vi "2D_density_plot_test.vi"() -> ()   [LabVIEW 2018]
uses:
  <vilib>/Heliosphere Research LLC/Advanced Plotting Toolkit/api_plotting/ContourFilledProperties.ctl
  <vilib>/Heliosphere Research LLC/Advanced Plotting Toolkit/properties/Colormap.ctl
  <vilib>/Heliosphere Research LLC/Advanced Plotting Toolkit/properties/Colormap_Map.ctl
  <vilib>/Heliosphere Research LLC/Advanced Plotting Toolkit/properties/Colormap_Scaling.ctl
  <vilib>/Heliosphere Research LLC/Advanced Plotting Toolkit/properties/Display.ctl
  <vilib>/Heliosphere Research LLC/Advanced Plotting Toolkit/api_plotting/ContourRange.ctl
  <vilib>/Heliosphere Research LLC/Advanced Plotting Toolkit/api_core/NewPlotType.ctl
  <vilib>/Heliosphere Research LLC/Advanced Plotting Toolkit/api_core/NewPlotScales.ctl
  <vilib>/Heliosphere Research LLC/Advanced Plotting Toolkit/api_plotting/ContourFilled_Automatic.vi
  <vilib>/Heliosphere Research LLC/Advanced Plotting Toolkit/Advanced Plotting Toolkit.lvlib
panel:
  in  "Contour Range":T1={"Min Level"=nan, "Max Level"=nan}
  in  "Log-transform?":bool=TRUE
  in  "Properties":T2={"Colormap"={"Map"=enum."Automatic", "Value Min"=nan, "Value Max"=nan, "Scaling"=enum."Default", "Reverse"=FALSE}, "Display"={"Alpha"=nan, "Z Order"=nan}}
  out "Picture":picture
  out "Image Display":T7(plugin-control)
  in  "Python file path":path
  out "alpha":dbl[](array[numeric])
  out "Y coord":dbl[](array[numeric])
  out "X coord":dbl[](array[numeric])
  out "error out":errorcluster
  in  "create index file? (T)":bool
  in  "File path":path
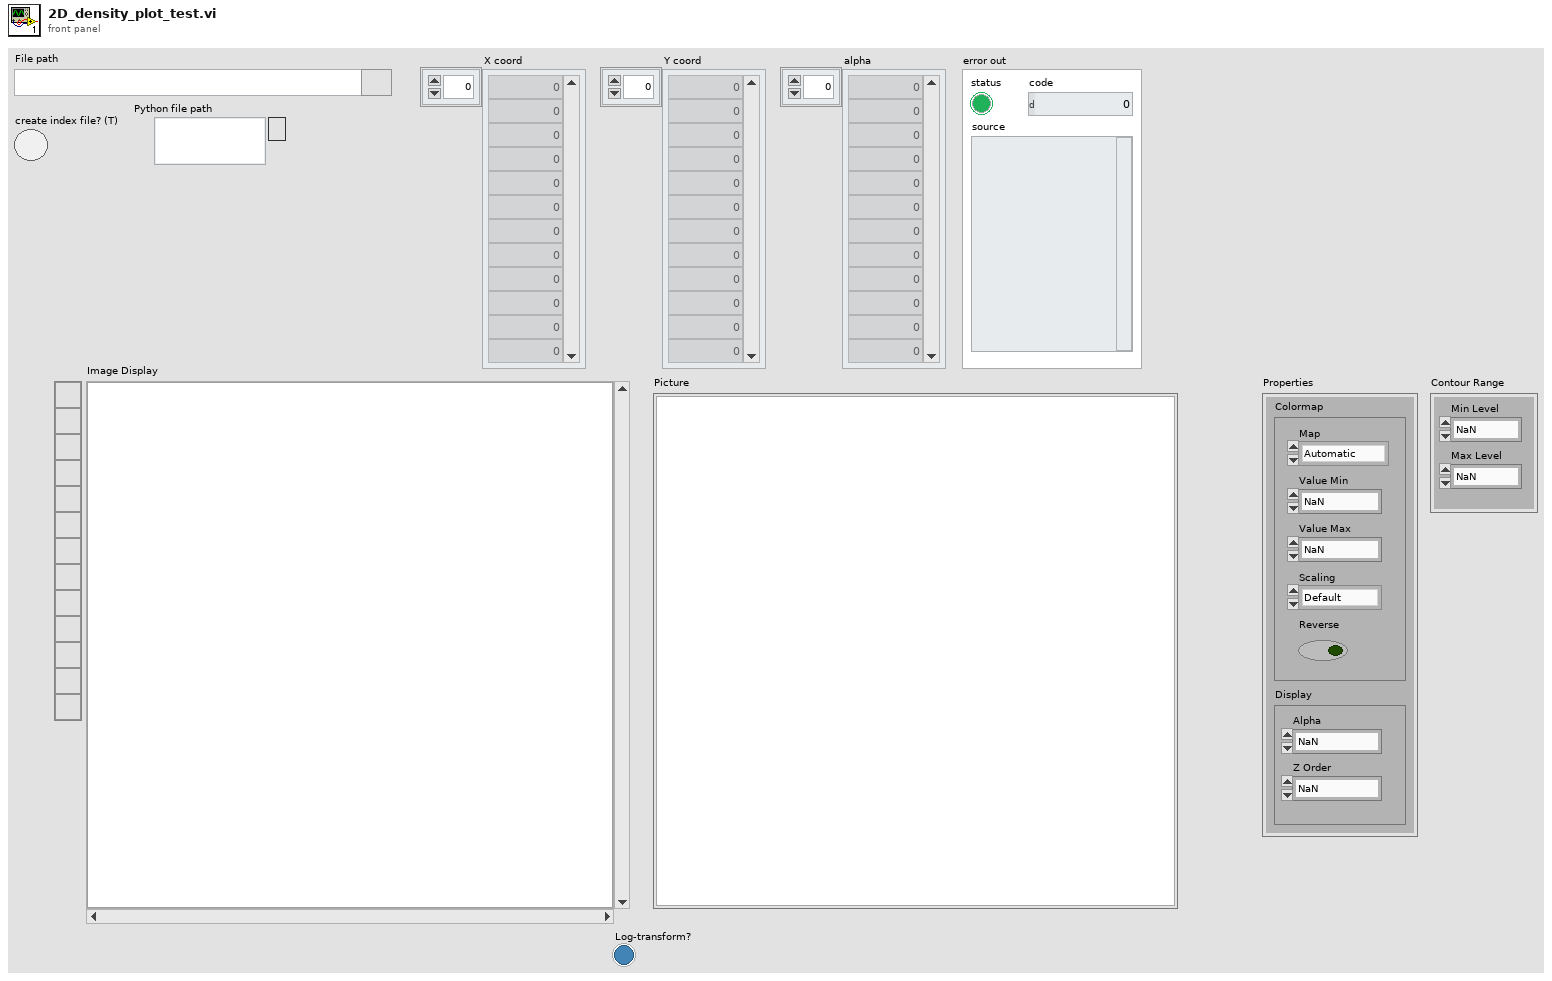
[diagram p1: front panel]
types:
  T1 = typedef "Advanced Plotting Toolkit.lvlib/ContourRange.ctl" = cluster{"Min Level":dbl, "Max Level":dbl}
  T2 = typedef "Advanced Plotting Toolkit.lvlib/ContourFilledProperties.ctl" = cluster{"Colormap":T3, "Display":T6}
  T3 = typedef "Advanced Plotting Toolkit.lvlib/Colormap.ctl" = cluster{"Map":T4, "Value Min":dbl, "Value Max":dbl, "Scaling":T5, "Reverse":bool}
  T4 = typedef "Advanced Plotting Toolkit.lvlib/Colormap_Map.ctl" = enum16{"Automatic", "Rainbow", "Hot and Cold", "White-Black", "White-Blue", "White-Green", "White-Red", "Fire", "Water", "Earth", "Air", "Pastel", "Banded", "Stepped"}
  T5 = typedef "Advanced Plotting Toolkit.lvlib/Colormap_Scaling.ctl" = enum16{"Default"}
  T6 = typedef "Advanced Plotting Toolkit.lvlib/Display.ctl" = cluster{"Alpha":dbl, "Z Order":dbl}
  T7 = typedef "IMAQ Image.ctl" = refnum<image>
  T8 = typedef "Advanced Plotting Toolkit.lvlib/NewPlotScales.ctl" = enum16{"Default", "Linear", "Log", "Symlog"}
  T9 = typedef "Advanced Plotting Toolkit.lvlib/NewPlotType.ctl" = enum16{"Rectangular Axes", "Polar Axes"}
  T10 = typedef "Image Type" = u32
  T11 = enum16{"big-endian, network order", "native, host order", "little-endian"}
  T12 = enum16{"open", "open or create", "create or replace", "create", "open (read-only)"}
  T13 = typedef "Advanced Plotting Toolkit.lvlib/PlotID.ctl" = i32
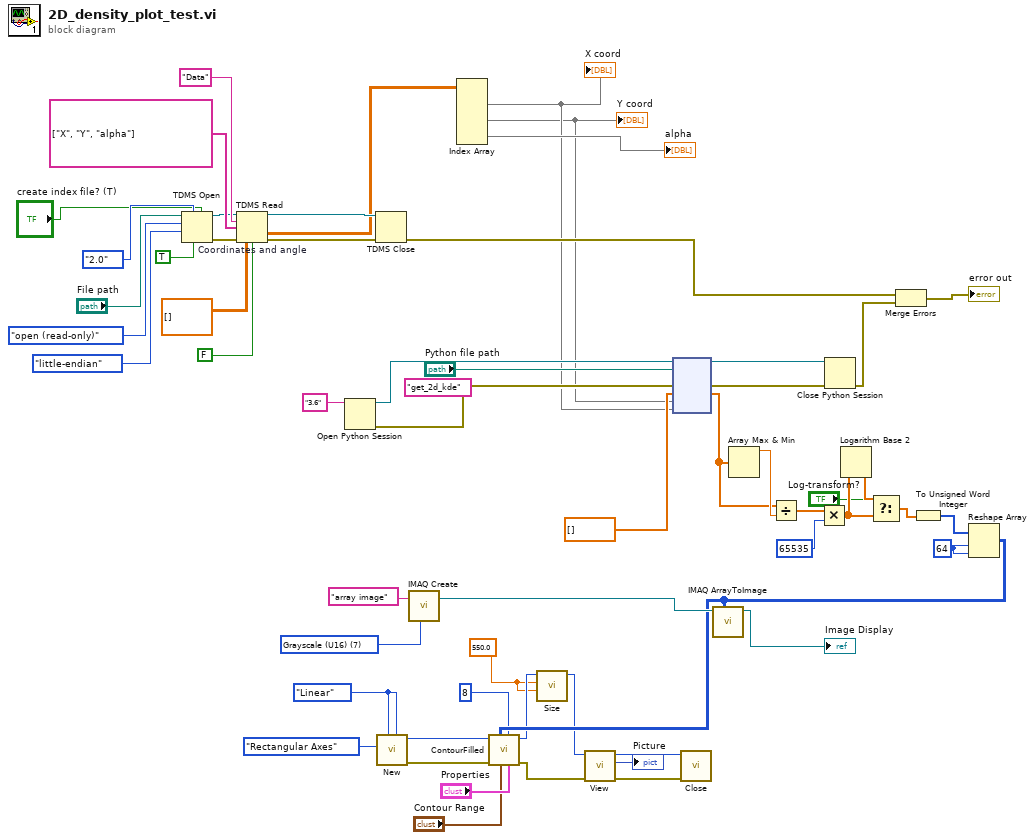
[diagram p0: block diagram]
diagram:
  w6 = 550.0 ("Width (pixels)")
  w18 = NewPlotScales."Linear" ("X Axis Scale")
  w29 = T10 7 items=["Grayscale (U8)", "Grayscale (I16)", "Grayscale (SGL)", "Complex (CSG)", "RGB (U32)", "HSL (U32)", "RGB (U64)", "Grayscale (U16)"] ("Image Type")
  w31 = 64 ("dimension size")
  n1 = TDMS Open(5:"create index file? (T)", 6:TRUE ("disable buffering? (T)"), 7:enum16{"1.0", "2.0"}."2.0" ("file format version (2.0)"), 9:T11."little-endian" ("byte order (2:little-endian)"), 10:T12."open (read-only)" ("operation (0:open)"), 11:"File path") -> (0:w47:errorcluster, 3:w48:refnum<k34>)  [unwired: 1 in]
  n2 = TDMS Read "Coordinates and angle"(0:w48, 5:"Data" ("group name in"), 7:string[] ["X", "Y", "alpha"] ("Columns Names"), 11:w47, 12:dbl[][] [], 13:FALSE ("return channels in file order? (F)")) -> (4:w46:refnum<k34>, 10:w43:dbl[][], 15:w45:errorcluster)  [unwired: 2 in, 3 out]
  n3 = Open Python Session(python version="3.6" ("Python version")) -> (session out=w42:refnum<k35>, error out=w40:errorcluster)  [unwired: 2 in]
  n4 = TDMS Close(8:w45, 11:w46) -> (0:w44:errorcluster)  [unwired: 1 out]
  n5 = call <vilib>:"New.vi"("Y Axis Scale"=w18, "X Axis Scale"=w18, "Plot Type"=NewPlotType."Rectangular Axes") -> ("error out"=w16:errorcluster, "Plot ID"=w17:T13)  [unwired: 7 in]
  n6 = call "IMAQ Create"("Image Name"="array image", "Image Type"=w29) -> ("New Image"=w26:T7)  [unwired: 3 in, 1 out]
  n7 = Index Array(array=w43) -> (element #1=w21:dbl[], element #2=w20:dbl[], element #3=→"alpha":dbl[])  [unwired: 6 in]
  "X coord" <- w21
  "Y coord" <- w20
  n8 = node(w42, "Python file path", "get_2d_kde" ("function name"), w40, dbl[] [], w20, w21) -> (w38:refnum<k35>, w37:errorcluster, w23:dbl[])  [unwired: 2 in, 2 out]
  n9 = Array Max & Min(array=w23) -> (max value=w28:dbl)  [unwired: 3 out]
  n10 = Divide(x=w23, y=w28) -> (x/y=w22:dbl[])
  n11 = Multiply(x=w22, y=65535 ("dimension size")) -> (x*y=w4:dbl[])
  n12 = Close Python Session(session in=w38, error in=w37) -> (11:w35:errorcluster)
  n13 = Logarithm Base 2(1:w4) -> (0:w3:dbl[])
  n14 = Select(t=w3, s="Log-transform?", f=w4) -> (s? t:f=w5:dbl[])
  n15 = Merge Errors(w44, w35) -> (→"error out":errorcluster)
  n16 = To Unsigned Word Integer(number=w5) -> (unsigned 16bit integer=w24:u16[])
  n17 = Reshape Array(w24, w31, w31) -> (w15:u16[][])
  n18 = call-poly <vilib>:"ContourFilled.vi"("Properties"="Properties", "Levels"=8, "Contour Range"="Contour Range", "Z Data"=w15, "error in (no error)"=w16, "Plot ID"=w17) -> ("error out"=w14:errorcluster, "Plot ID Out"=w8:T13)  [unwired: 4 in]
  n19 = call <vilib>:"Size.vi"("Height (pixels)"=w6, "Width (pixels)"=w6, "Plot ID"=w8) -> ("Plot ID Out"=w7:T13)  [unwired: 7 in, 1 out]
  n20 = call <vilib>:"View.vi"("error in (no error)"=w14, "Plot ID"=w7) -> ("error out"=w12:errorcluster, "Picture"=→"Picture":picture, "Plot ID Out"=w13:T13)  [unwired: 7 in]
  n21 = call <vilib>:"Close.vi"("error in (no error)"=w12, "Plot ID"=w13) -> ()  [unwired: 9 in, 1 out]
  n22 = call "IMAQ ArrayToImage"("Image Pixels (U16)"=w15, "Image"=w26) -> ("Image Out"=→"Image Display":T7)  [unwired: 8 in, 1 out]
